vi "Current Y Value Write.vi"(4 "error in (no error)":errorcluster, 5 "Value":dbl, 6 "Container State":T2, 7 "Display State In":T1={"Measure ?"=[], "Direction"=[], "Loop ?"={"Start"=0, "Finish"=2}, "Storage Location"=[], "Show Current Location"=FALSE, "Current Location"=0, "Show y=0"=FALSE, "Program"=[], "Index"=0, "Average During Loop ?"=FALSE, "# of Loops"=1, "Loop Control"={0, 2}, "Units"="", "Digits"=0, "Significant Figures (F) or DP (T)"=FALSE, "Rate Mode"=FALSE, "Current Y value"=0.0, "Initial Value"=0.0} {"# of Loops" min=1 step=1; "Index" min=0 step=1; "Program"."Step" min=0.001 max=80.0 step=0.001 format="%.2f"; "Program"."Target" format="%.2f"}) -> (0 "error out":errorcluster, 3 "Display State Out":T1={"Measure ?"=[], "Direction"=[], "Loop ?"={"Start"=0, "Finish"=2}, "Storage Location"=[], "Show Current Location"=FALSE, "Current Location"=0, "Show y=0"=FALSE, "Program"=[], "Index"=0, "Average During Loop ?"=FALSE, "# of Loops"=1, "Loop Control"={0, 2}, "Units"="", "Digits"=0, "Significant Figures (F) or DP (T)"=FALSE, "Rate Mode"=FALSE, "Current Y value"=0.0, "Initial Value"=0.0} {"# of Loops" min=1 step=1; "Index" min=0 step=1; "Program"."Step" min=0.001 max=80.0 step=0.001 format="%.2f"; "Program"."Target" format="%.2f"})   [LabVIEW 2018, in "Multi Segment Waveform.xctl"]
uses:
  Multi Segment Waveform.xctl
  <vilib>/_xctls/Container State.ctl
  State.ctl
  <vilib>/_xctls/XControlSupport.lvlib
panel:
  # "Replace the Value Control below with a Control of desired type.\nDo not remove this Control or the others from the connector pane.\nDo not change the connector pane pattern.\nThe Value control should always be the third terminal from top on the input side in the connector pane."
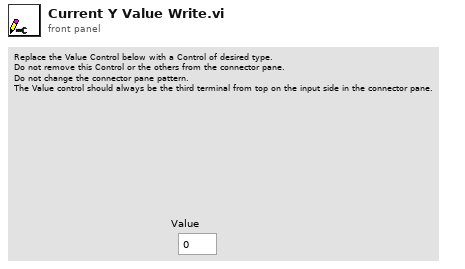
[diagram p1: front panel]
types:
  T1 = typedef "Multi Segment Waveform.xctl/State.ctl" = cluster{"Measure ?":bool[], "Direction":bool[], "Loop ?":cluster{"Start":i32, "Finish":i32}, "Storage Location":i32[], "Show Current Location":bool, "Current Location":i32, "Show y=0":bool, "Program":cluster{"Target":dbl, "Step":dbl, "Measure ?":bool}[], "Index":i32, "Average During Loop ?":bool, "# of Loops":u32, "Loop Control":cluster{i32, i32}, "Units":string, "Digits":i32, "Significant Figures (F) or DP (T)":bool, "Rate Mode":bool, "Current Y value":dbl, "Initial Value":dbl}
  T2 = typedef "XControlSupport.lvlib/Container State.ctl" = cluster{"Indicator?":bool, "Run Mode?":bool, " Refnum":refnum<vi>}
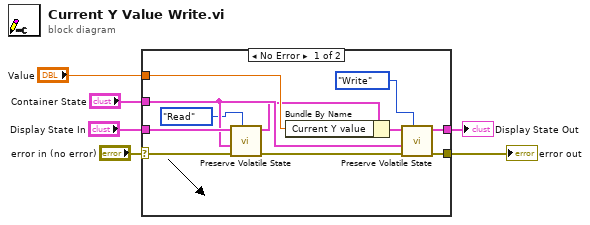
[diagram p0: block diagram]
diagram:
  n1 = case shown="No Error" "error in (no error)" {
    selector: "error in (no error)" -> [w15 w19]
    tunnel: "Value" -> [w17 _]
    tunnel: "Display State In" -> [w16 w18]
    tunnel: "Container State" -> [w14 _]
    tunnel: [w12 w19] -> w2
    tunnel: [w9 w18] -> w1
    frame No Error {
      n2 = call "Preserve Volatile State.vi"("Operation"=enum16{"Read", "Write", "Update From Data"}."Read", "error in (no error)"=w15, "Container State"=w14, "Waveform State In"=w16) -> ("error out"=w13:errorcluster, "Waveform State Out"=w11:T1)  [unwired: 1 in, 5 out]
      n3 = Bundle By Name(cluster=w11, "Current Y value"=w17) -> (w10:T1)
      n4 = call "Preserve Volatile State.vi"("Operation"=enum16{"Read", "Write"}."Write", "error in (no error)"=w13, "Container State"=w14, "Waveform State In"=w10) -> ("error out"=w12:errorcluster, "Waveform State Out"=w9:T1)  [unwired: 1 in, 5 out]
    }
    frame Error {
    }
  }
  "error out" <- w2
  "Display State Out" <- w1
